vi "Read Log File.vi"(8 "error in":errorcluster, 11 "Path":path) -> (0 "error out":errorcluster, 3 "File Data":string[](array[string]))   [LabVIEW 2020, in "SECS Bridge.lvlib"]
uses:
  SECS Bridge.lvlib
  SECS Communication/HSMS Class/Notifier Data.ctl
  SECS Communication/HSMS Class/Notifier Type.ctl
  SECS Communication/HSMS Class/HSMS Class.lvclass
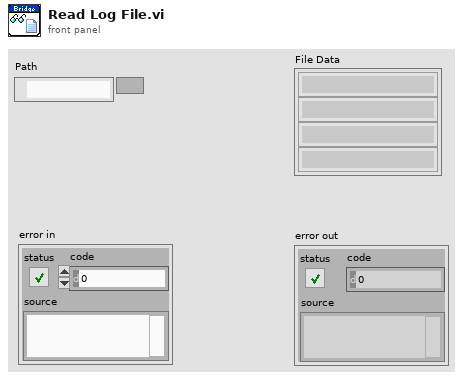
[diagram p1: front panel]
types:
  T1 = typedef "SECS Communication.lvlib/HSMS Class.lvclass/Notifier Data.ctl" = cluster{"Notifier Type":T2, "Data":variant, "Time":timestamp}
  T2 = typedef "SECS Communication.lvlib/HSMS Class.lvclass/Notifier Type.ctl" = enum16{"TCPIP Connect", "TCPIP Disconnect", "Receive Message", "Send Message", "T3 Timeout", "T6 Timeout", "T7 Timeout", "Error", "Stop"}
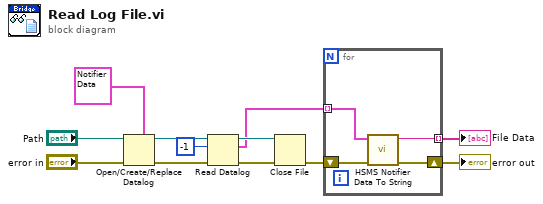
[diagram p0: block diagram]
diagram:
  n1 = Open/Create/Replace Datalog(5:T1 {"Notifier Type"=enum."Receive Message", "Data"=variant, "Time"=timestamp(0 s since 1904-01-01)} ("Notifier Data"), 8:"error in", 11:"Path") -> (0:w12:errorcluster, 3:w7:refnum<k1>)  [unwired: 3 in, 1 out]
  n2 = Read Datalog(4:w12, 6:-1 ("count (1)"), 7:w7) -> (0:w11:errorcluster, 2:w4:T1[], 3:w6:refnum<k1>)
  n3 = Close File(refnum=w6, error in=w11) -> (error out=w3:errorcluster)  [unwired: 1 out]
  n4 = for {
    tunnel: w4 -> [w15] mode=indexing
    shift-right: [w14] -> w1
    shift-left: w3 -> [w16]
    tunnel: [w13] -> w2 mode=indexing
    n5 = call "HSMS Notifier Data To String.vi"("error in (no error)"=w16, "Notifier Data"=w15) -> ("error out"=w14:errorcluster, "String"=w13:string)  [unwired: 8 in]
  }
  "error out" <- w1
  "File Data" <- w2
